vi "repeatcalc-for.vi"() -> ()   [LabVIEW 2009]
panel:
  out "x^2":i32
  in  "Numeric":i32
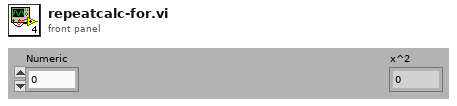
[diagram p1: front panel]
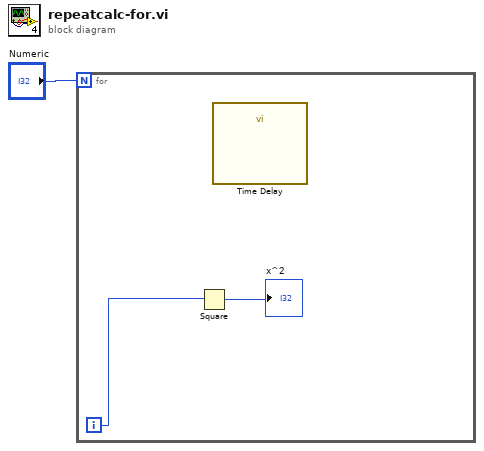
[diagram p0: block diagram]
diagram:
  n1 = for {
    N: "Numeric" -> [_]
    i -> [w3]
    n2 = Square(x=w3) -> (x^2=→"x^2":i32)
    n3 = call "Time Delay"() -> ()  [unwired: 11 in, 1 out]
  }
